vi "Motors Decipher Status.vi"(1 "OS":i32) -> (0 "Status":string)   [LabVIEW 2018]
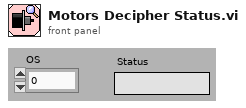
[diagram p1: front panel]
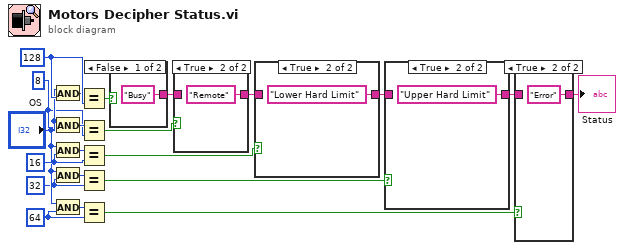
[diagram p0: block diagram]
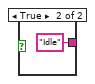
[diagram p6: hidden frame]
diagram:
  w2 = 64 ("y")
  w5 = 32 ("y")
  w20 = 16 ("y")
  w8 = 8 ("y")
  w17 = 128 ("y")
  n1 = And(x="OS", y=w17) -> (x .and. y?=w16:i32)
  n2 = And(x="OS", y=w8) -> (x .and. y?=w9:i32)
  n3 = And(x="OS", y=w20) -> (x .and. y?=w19:i32)
  n4 = And(x="OS", y=w5) -> (x .and. y?=w6:i32)
  n5 = And(x="OS", y=w2) -> (x .and. y?=w3:i32)
  n6 = Equal?(x=w16, y=w17) -> (x = y?=w18:bool)
  n7 = Equal?(x=w9, y=w8) -> (x = y?=w7:bool)
  n8 = Equal?(x=w19, y=w20) -> (x = y?=w21:bool)
  n9 = Equal?(x=w6, y=w5) -> (x = y?=w4:bool)
  n10 = Equal?(x=w3, y=w2) -> (x = y?=w1:bool)
  n11 = case shown="False" w18 {
    tunnel: ["Busy" "Idle"] -> w10
    frame False {
    }
    frame True {
    }
  }
  n12 = case shown="True" w7 {
    tunnel: w10 -> [w24 _]
    tunnel: [w24 "Remote"] -> w11
    frame False {
    }
    frame True {
    }
  }
  n13 = case shown="True" w21 {
    tunnel: w11 -> [w26 _]
    tunnel: [w26 "Lower Hard Limit"] -> w12
    frame False {
    }
    frame True {
    }
  }
  n14 = case shown="True" w4 {
    tunnel: w12 -> [w28 _]
    tunnel: [w28 "Upper Hard Limit"] -> w14
    frame False {
    }
    frame True {
    }
  }
  n15 = case shown="True" w1 {
    tunnel: w14 -> [w30 _]
    tunnel: [w30 "Error"] -> w15
    frame False {
    }
    frame True {
    }
  }
  "Status" <- w15
